vi "Add Project Item.vi"(8 "error in (no error)":errorcluster, 10 "Folder Location Ref":refnum<vi>, 11 "EST Bidirectional Sensor in":refnum<class "EST Bidirectional Sensor.lvclass">) -> (0 "error out":errorcluster, 3 "EST Bidirectional Sensor out":refnum<class "EST Bidirectional Sensor.lvclass">)   [LabVIEW 2015, in "EST Bidirectional Sensor.lvclass"]
uses:
  EST Bidirectional Sensor.lvclass
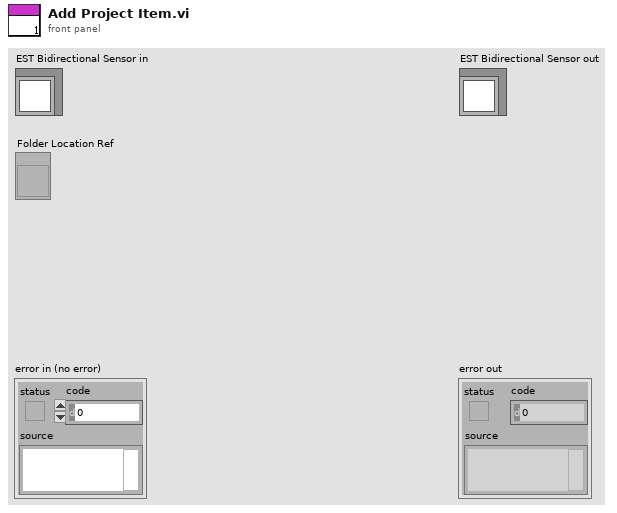
[diagram p1: front panel]
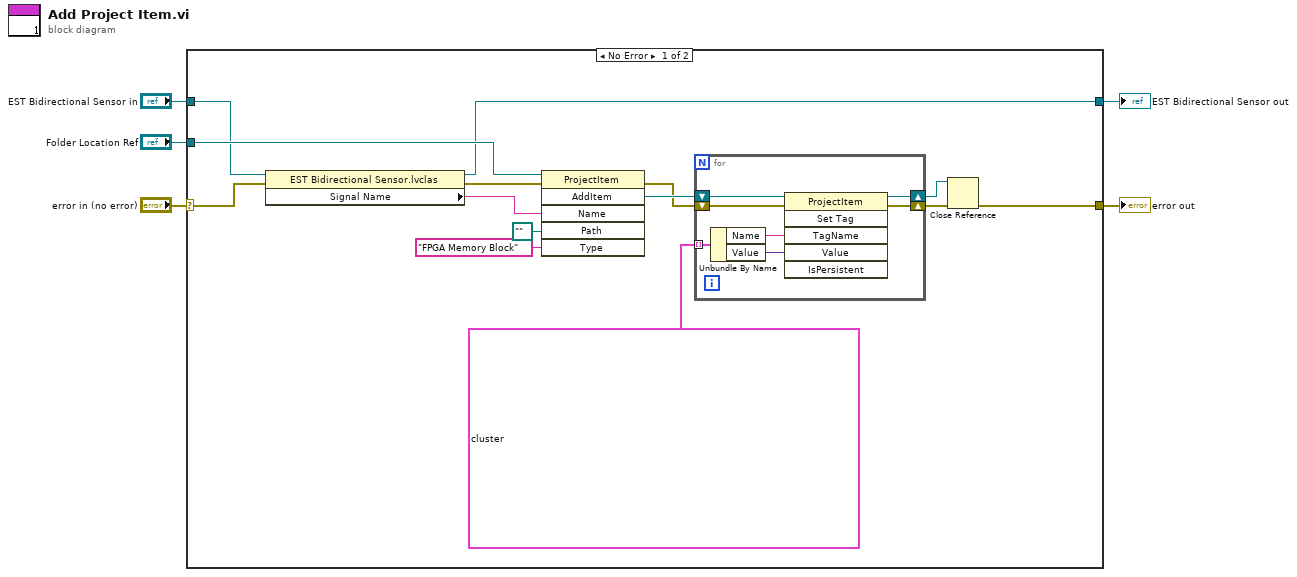
[diagram p0: block diagram]
diagram:
  n1 = case shown="No Error" "error in (no error)" {
    selector: "error in (no error)" -> [w9 w27]
    tunnel: "Folder Location Ref" -> [w12 _]
    tunnel: "EST Bidirectional Sensor in" -> [w11 w28]
    tunnel: [w7 w28] -> w2
    tunnel: [w6 w27] -> w1
    frame No Error {
      n2 = property class="EST Bidirectional Sensor.lvclas"(reference=w11, error in=w9) -> (reference out=w7:refnum<class "EST Bidirectional Sensor.lvclass">, error out=w8:errorcluster, "Signal Name"=w10:string)
      n3 = invoke class="ProjectItem" method="AddItem"(reference=w12, error in=w8, "Name"=w10, "Path"=path "", "Type"="FPGA Memory Block") -> (error out=w16:errorcluster, "AddItem"=w18:refnum<vi>)  [unwired: 1 in, 4 out]
      n4 = for {
        shift-right: [w21] -> w14
        shift-left: w16 -> [w25]
        tunnel: cluster{"Name":string, "Value":variant}[] [{"Name"="FPGA.PersistentID", "Value"=variant(string "{CD7EB185-1A87-4E78-8C08-5D9A1491F439}")}, {"Name"="fullEmulation", "Value"=variant(bool TRUE)}, {"Name"="Memory Latency", "Value"=variant(u32 1)}, {"Name"="Multiple Clock Domains", "Value"=variant(bool FALSE)}, {"Name"="NI.LV.FPGA.CompileConfigString", "Value"=variant(string "Actual Number of Elements=1024;ReadArbs=2;WriteArbs=2;Implementation=2;DataType=100080000000000100094006000355313600010000000000000000;InitDataHash=;DRAM Selection=DramBank0;DRAM Max Outstanding Requests=64;DRAM Include Byte Enables=FALSE;DRAM Grant Time=50;Interface Configuration=Read A-Write B;Multiple Clock Domains=FALSE;Memory Latency=1")}, {"Name"="NI.LV.FPGA.MEMORY.ActualNumberOfElements", "Value"=variant(u32 1024)}, {"Name"="NI.LV.FPGA.MEMORY.DataWidth", "Value"=variant(u32 6)}, {"Name"="NI.LV.FPGA.MEMORY.DramIncludeByteEnables", "Value"=variant(bool FALSE)}, {"Name"="NI.LV.FPGA.MEMORY.DramMaxOutstandingRequests", "Value"=variant(i32 64)}, {"Name"="NI.LV.FPGA.MEMORY.DramSelection", "Value"=variant(string "DramBank0")}, {"Name"="NI.LV.FPGA.MEMORY.Init", "Value"=variant(bool FALSE)}, {"Name"="NI.LV.FPGA.MEMORY.InitData", "Value"=variant(string "")}, {"Name"="NI.LV.FPGA.MEMORY.InitVIPath", "Value"=variant(string "")}, {"Name"="NI.LV.FPGA.MEMORY.InterfaceAArbitration", "Value"=variant(u32 2)}, {"Name"="NI.LV.FPGA.MEMORY.InterfaceBArbitration", "Value"=variant(u32 2)}, {"Name"="NI.LV.FPGA.MEMORY.InterfaceConfig", "Value"=variant(u32 0)}, {"Name"="NI.LV.FPGA.MEMORY.RequestedNumberOfElements", "Value"=variant(u32 1024)}, {"Name"="NI.LV.FPGA.MEMORY.Type", "Value"=variant(u32 2)}, {"Name"="NI.LV.FPGA.ScriptConfigString", "Value"=variant(string "Actual Number of Elements=1024;ReadArbs=2;WriteArbs=2;Implementation=2;DataType=100080000000000100094006000355313600010000000000000000;InitDataHash=;DRAM Selection=DramBank0;DRAM Max Outstanding Requests=64;DRAM Include Byte Enables=FALSE;DRAM Grant Time=50;Interface Configuration=Read A-Write B;Multiple Clock Domains=FALSE;Memory Latency=1Persist Memory ValuesTRUE;")}, {"Name"="NI.LV.FPGA.Valid", "Value"=variant(bool TRUE)}, {"Name"="NI.LV.FPGA.Version", "Value"=variant(i32 10)}, {"Name"="Type Descriptor", "Value"=variant(string "100080000000000100094006000355313600010000000000000000")}] ("Array 2") -> [w24] mode=indexing
        shift-right: [w20] -> w15
        shift-left: w18 -> [w26]
        n5 = Unbundle By Name(w24) -> ("Name"=w23:string, "Value"=w22:variant)
        n6 = invoke class="ProjectItem" method="Set Tag"(reference=w26, error in=w25, "TagName"=w23, "Value"=w22) -> (reference out=w20:refnum<vi>, error out=w21:errorcluster)  [unwired: 2 in, 4 out]
      }
      n7 = Close Reference(reference=w15, error in (no error)=w14) -> (error out=w6:errorcluster)
    }
    frame Error {
    }
  }
  "error out" <- w1
  "EST Bidirectional Sensor out" <- w2
